vi "DIO_Read8.vi"() -> ()   [LabVIEW 2012]
doc: "This VI can be used to read a single byte from an ACCESS USB-DIO card."
uses:
  Windows/System32/AIOUSB.dll
panel:
  out "error out":errorcluster
  in  "error in (no error)":errorcluster
  out "Return Value":u32
  out "Reading":u8
  in  "Byte Index":u32
  in  "DeviceIndex":u32 max=32
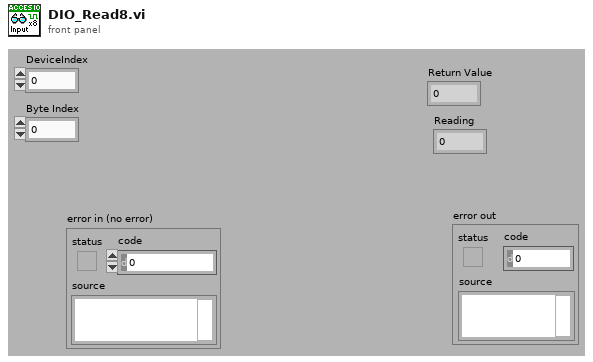
[diagram p1: front panel]
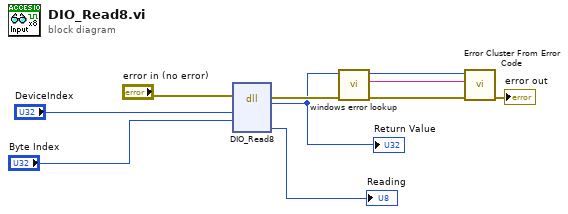
[diagram p0: block diagram]
diagram:
  n1 = dll-call lib="C:/Windows/System32/AIOUSB.dll" fn="DIO_Read8"(error in="error in (no error)", "DeviceIndex"="DeviceIndex", "ByteIndex"="Byte Index") -> (error out=w4:errorcluster, w1:u32, "pBuffer"=→"Reading":u8)  [unwired: 5 in, 1 out]
  "Return Value" <- w1
  n2 = call "windows error lookup.vi"("error in (no error)"=w4, "Error Code"=w1) -> ("error out"=w5:errorcluster, "error message (\"\")"=w7:string)  [unwired: 8 in]
  n3 = call <vilib>:"Error Cluster From Error Code.vi"("error in (no error)"=w5, "error message (\"\")"=w7, "error code (0)"=w1) -> ("error out"=→"error out":errorcluster)  [unwired: 6 in]
